vi "SQL写入 - 穿管.vi"(5 "TestMessage":string, 11 "error in (no error)":errorcluster caption="错误输入（无错误）") -> (15 "error out":errorcluster caption="错误输出")   [LabVIEW 2017]
panel:
  out "当前日期时间":string
  out "连接的字符串":string
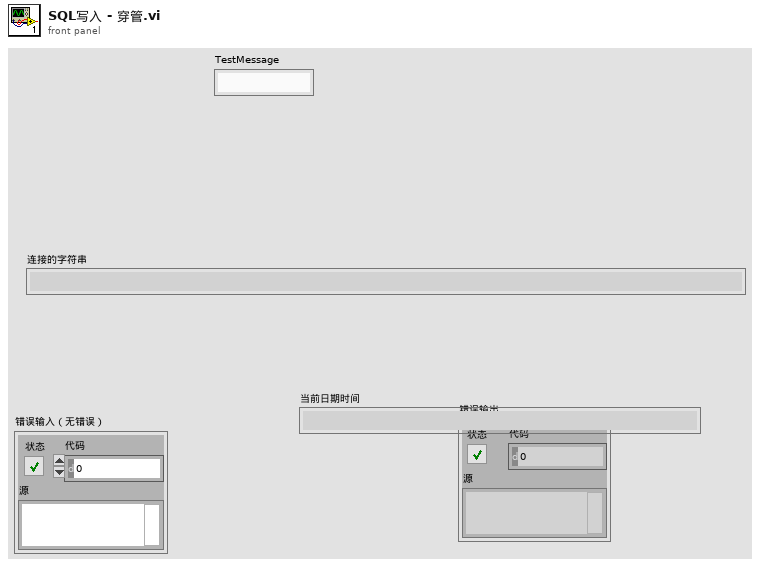
[diagram p1: front panel]
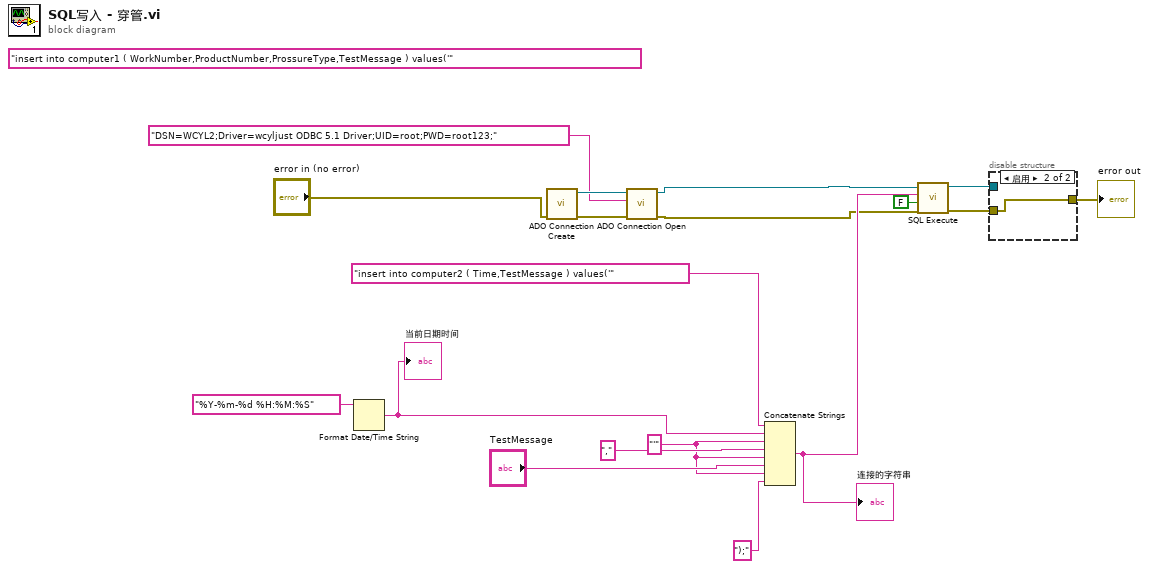
[diagram p0: block diagram]
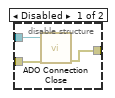
[diagram p2: hidden frame]
diagram:
  (unwired) "insert into computer1 ( WorkNumber,ProductNumber,ProssureType,TestMessage ) values('" ("Command Text")
  w15 = "'" ("字符串")
  n1 = Format Date/Time String(time format string (%c)="%Y-%m-%d %H:%M:%S" ("时间格式字符串(%c)")) -> (date/time string=w1:string)  [unwired: 2 in]
  "当前日期时间" <- w1
  n2 = call <userlib>:"ADO Connection Create.vi"("error in (no error)"="error in (no error)") -> ("error out"=w13:errorcluster, "ADODB._Connection Out"=w14:refnum<k7>)  [unwired: 9 in]
  n3 = call <userlib>:"ADO Connection Open.vi"("error in (no error)"=w13, "ConnectionString"="DSN=WCYL2;Driver=wcyljust ODBC 5.1 Driver;UID=root;PWD=root123;", "ADODB._Connection In"=w14) -> ("error out"=w4:errorcluster, "ADODB._Connection Out"=w5:refnum<k7>)  [unwired: 7 in]
  n4 = Concatenate Strings("insert into computer2 ( Time,TestMessage ) values('" ("Command Text"), w1, w15, "," ("字符串"), w15, "TestMessage", w15, ");" ("字符串")) -> (w11:string)
  "连接的字符串" <- w11
  n5 = call <userlib>:"SQL Execute.vi"("error in (no error)"=w4, "Return Data (T)"=FALSE, "Command Text"=w11, "ADODB._Connection In"=w5) -> ("error out"=w9:errorcluster, "ADODB._Connection Out"=w10:refnum<k7>)  [unwired: 4 in, 2 out]
  n6 = disable-structure shown="启用" {
    disable-tunnel: w10 -> [w21 _]
    disable-tunnel: w9 -> [w20 w22]
    disable-tunnel: [w19 w22] -> w7
    frame Disabled {
      n7 = call <userlib>:"ADO Connection Close.vi"("error in (no error)"=w20, "ADODB._Connection In"=w21) -> ("error out"=w19:errorcluster)  [unwired: 8 in, 1 out]
    }
    frame Enabled {
    }
  }
  "error out" <- w7
